vi "Setup file.vi"(5 "Stimulus":T1 {"noise freq hi" min=0.0 step=0.5; "noise freq lo" min=0.0 step=0.5; "noiseamp end" min=0.0 step=0.5; "noiseamp start" min=0.0 step=0.5}, 7 "motor":dbl[](array[numeric]), 8 "error in (no error)":errorcluster, 10 "Sampling data":T5={"Channels"=[], "Sampling freq"=0.0, "Output freq"=0.0, "Update freq"=0.0, "Steps per rev"=0, "Counts per rev"=0, "Amplifier"="", "Motor driver"="", "Step bit"=0, "Max speed"=0.0, "Max accel"=0.0, "Pos gain"=0.0, "Vel gain"=0.0, "counter"="Dev1/ctr0"} {"Channels"."Hi cutoff" items=["500"=500.0, "1k"=1000.0, "5k"=5000.0, "10k"=10000.0, "20k"=20000.0]; "Channels"."Lo cutoff" items=["0.1"=0.1, "1"=1.0, "10"=10.0, "100"=100.0, "300"=300.0]; "Channels"."Gain" items=["x100"=100, "x1000"=1000, "x10000"=10000]}, 11 "selected path":path) -> (0 "error out":errorcluster, 2 "Sampling data out":T5={"Channels"=[], "Sampling freq"=0.0, "Output freq"=0.0, "Update freq"=0.0, "Steps per rev"=0, "Counts per rev"=0, "Amplifier"="", "Motor driver"="", "Step bit"=0, "Max speed"=0.0, "Max accel"=0.0, "Pos gain"=0.0, "Vel gain"=0.0, "counter"="Dev1/ctr0"} {"Channels"."Hi cutoff" items=["500"=500.0, "1k"=1000.0, "5k"=5000.0, "10k"=10000.0, "20k"=20000.0]; "Channels"."Lo cutoff" items=["0.1"=0.1, "1"=1.0, "10"=10.0, "100"=100.0, "300"=300.0]; "Channels"."Gain" items=["x100"=100, "x1000"=1000, "x10000"=10000]}, 3 "file refs":T3 {"file" format="%.0x"}, 4 "path out":path)   [LabVIEW 2013]
uses:
  Sampling info.ctl
  Channel.ctl
  File refs.ctl
  <vilib>/addons/h5labview2/base/hid_t.ctl
  Stimulus.ctl
  Stimulus type.ctl
  <vilib>/addons/h5labview2/file/H5Fmode.ctl
  <vilib>/addons/h5labview2/file/H5F.lvlib
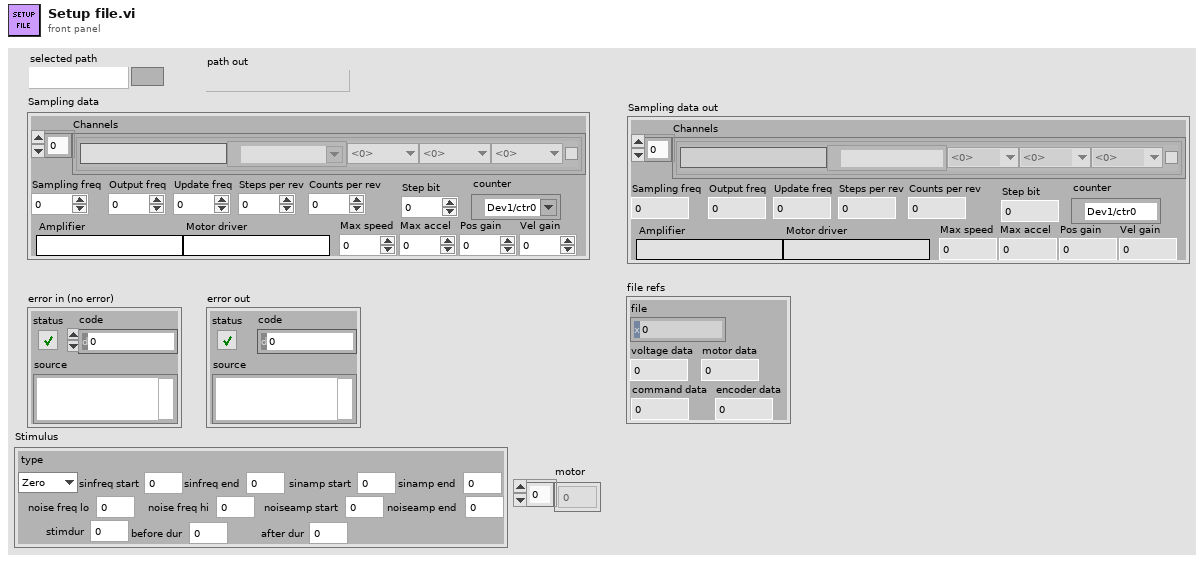
[diagram p1: front panel]
types:
  T1 = typedef "Stimulus.ctl" = cluster{"type":T2, "sinfreq start":dbl, "sinfreq end":dbl, "sinamp start":dbl, "sinamp end":dbl, "noise freq lo":dbl, "noise freq hi":dbl, "noiseamp start":dbl, "noiseamp end":dbl, "stimdur":dbl, "before dur":dbl, "after dur":dbl}
  T2 = typedef "Stimulus type.ctl" = enum16{"Zero", "Sine", "Frequency sweep", "Two frequency", "Amplitude sweep"}
  T3 = typedef "File refs.ctl" = cluster{"file":T4, "voltage data":i32, "motor data":i32, "command data":i32, "encoder data":i32}
  T4 = typedef "hid_t.ctl" = i32
  T5 = typedef "Sampling info.ctl" = cluster{"Channels":T6[], "Sampling freq":dbl, "Output freq":dbl, "Update freq":dbl, "Steps per rev":i32, "Counts per rev":i32, "Amplifier":string, "Motor driver":string, "Step bit":u8, "Max speed":dbl, "Max accel":dbl, "Pos gain":dbl, "Vel gain":dbl, "counter":tag}
  T6 = typedef "Channel.ctl" = cluster{"Name":string, "Chan":tag, "Gain":u16, "Lo cutoff":dbl, "Hi cutoff":dbl, "Notch":bool}
  T7 = typedef "H5F.lvlib/H5Fmode.ctl" = enum16{"read-only", "read-write", "overwrite", "create new", "open or create"}
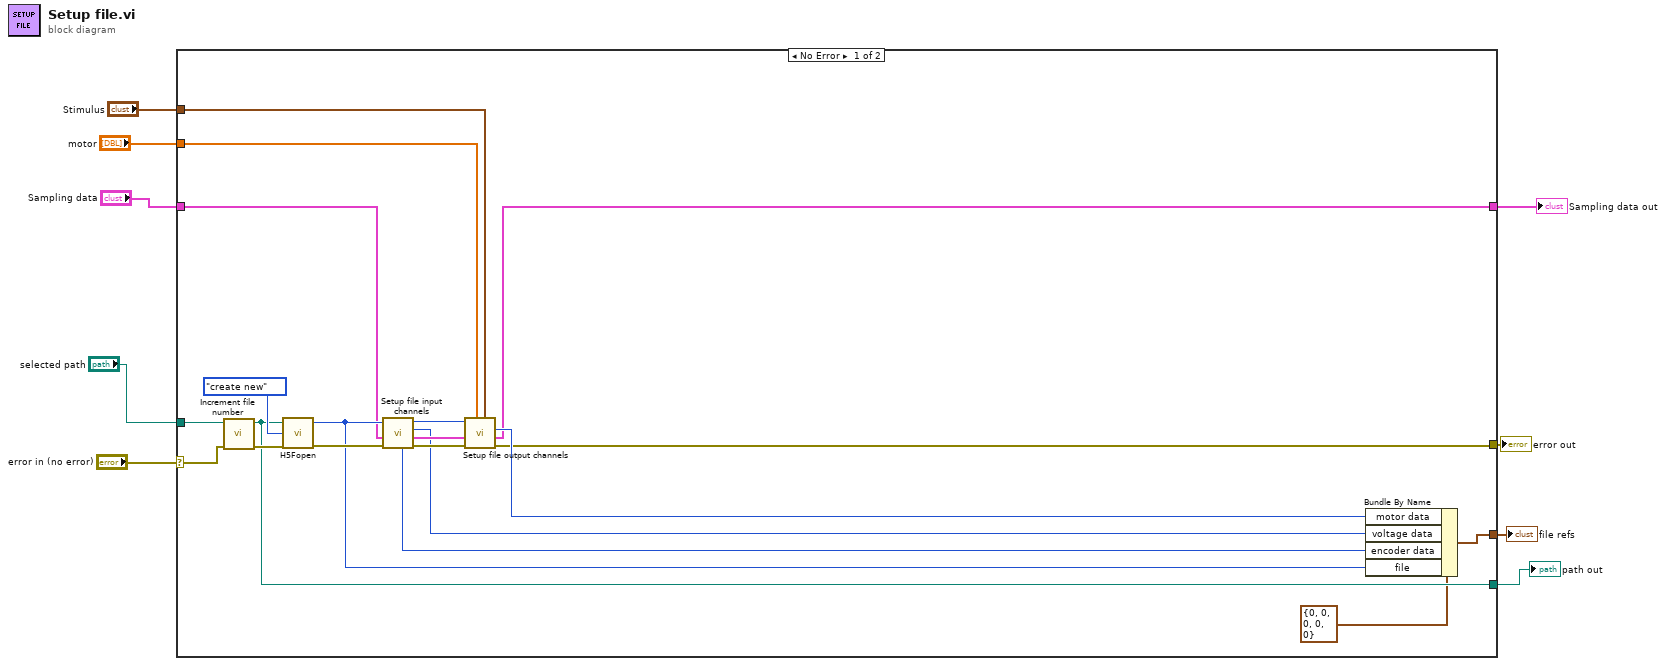
[diagram p0: block diagram]
diagram:
  n1 = case shown="No Error" "error in (no error)" {
    selector: "error in (no error)" -> [w28 w31]
    tunnel: "selected path" -> [w29 _]
    tunnel: "Sampling data" -> [w14 w30]
    tunnel: [w15 w31] -> w6
    tunnel: [w13 w30] -> w5
    tunnel: [w25 _] -> w3
    tunnel: [w24 _] -> w4
    tunnel: "motor" -> [w11 _]
    tunnel: "Stimulus" -> [w10 _]
    frame No Error {
      n2 = call "Increment file number.vi"("error in"=w28, "path"=w29) -> ("error out"=w27:errorcluster, "path out"=w24:path)  [unwired: 8 in]
      n3 = call <vilib>:"H5Fopen.vi"("error in (no error)"=w27, "mode (read-only)"=H5Fmode."create new", "path"=w24) -> ("error out"=w22:errorcluster, "ref out"=w18:T4)  [unwired: 1 in]
      n4 = call "Setup file input channels.vi"("error in"=w22, "Sampling data"=w14, "file ref in"=w18) -> ("error out"=w20:errorcluster, "Sampling data out"=w19:T5, "dset ref"=w17:i32, "file ref out"=w21:T4, "encoder dset"=w12:i32)  [unwired: 4 in]
      n5 = call "Setup file output channels.vi"("Stimulus"=w10, "motor"=w11, "error in"=w20, "Sampling data"=w19, "file ref in"=w21) -> ("error out"=w15:errorcluster, "Sampling data out"=w13:T5, "dset ref"=w16:i32)  [unwired: 3 in, 1 out]
      n6 = Bundle By Name(cluster=T3 {"file"=0, "voltage data"=0, "motor data"=0, "command data"=0, "encoder data"=0} ("file refs 2"), "motor data"=w16, "voltage data"=w17, "encoder data"=w12, "file"=w18) -> (w25:T3)
    }
    frame Error {
    }
  }
  "error out" <- w6
  "Sampling data out" <- w5
  "file refs" <- w3
  "path out" <- w4
